vi "get supported types.vi"(8 "error in":errorcluster, 11 "Asynchronous Component Configuration In":refnum<class "asynchronous execution module configuration.lvclass">) -> (0 "error out":errorcluster, 2 "supported types":T1[](array[typedef]), 3 "Asynchronous Component Configuration Out":refnum<class "asynchronous execution module configuration.lvclass">)   [LabVIEW 2013, in "asynchronous execution module configuration.lvclass"]
doc: "Provides an interface for determining the targets supported by a given configuration/runtime class pairing. This should be overridden by any useful child class."
uses:
  asynchronous execution module configuration.lvclass
  <vilib>/NI/Tag Bus/tag/Data Type.ctl
  asynchronous execution module configuration.lvclass/asynchronous execution module configuration.ctl
  <vilib>/NI/Tag Bus Module Framework/module configuration/TBM module configuration.lvclass
  <vilib>/NI/Tag Bus/tag/tag descriptor.lvclass
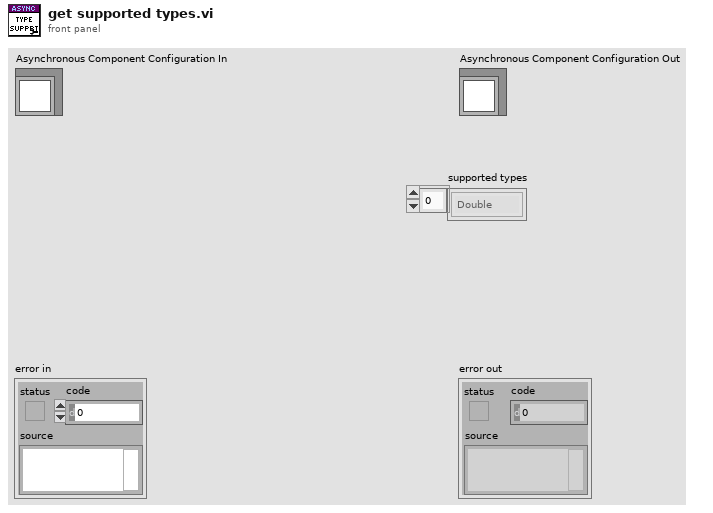
[diagram p1: front panel]
types:
  T1 = typedef "tag bus.lvlib/tag descriptor.lvclass/Data Type.ctl" = enum16{"Double", "Single", "I64", "I32", "I16", "I8", "U64", "U32", "U16", "U8", "Boolean", "String", "Array of Double", "Array of Single", "Array of I64", "Array of I32", "Array of I16", "Array of I8", "Array of U64", "Array of U32", "Array of U16", "Array of U8", "Array of Boolean", "Array of String"}
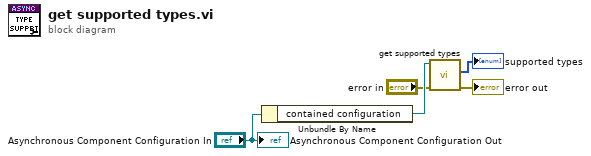
[diagram p0: block diagram]
diagram:
  n1 = Unbundle By Name("Asynchronous Component Configuration In") -> ("contained configuration"=w4:refnum<class "TBM module configuration.lvclass">)
  n2 = call-dynamic "get supported types.vi"("error in"="error in", "module configuration in"=w4) -> ("error out"=→"error out":errorcluster, "supported types"=→"supported types":T1[])  [unwired: 7 in, 1 out]
  "Asynchronous Component Configuration Out" <- "Asynchronous Component Configuration In"
